vi "GetBandCalculation.vi"(8 "error in (no error)":errorcluster, 11 "Properties In":T2[](array[typedef])) -> (0 "error out":errorcluster, 2 "Calculation":T1, 3 "Properties Out":T2[](array[typedef]))   [LabVIEW 2017, in "AnalysisHelper.lvlib"]
uses:
  <vilib>/addons/InsightCM/Utilities/Analysis/Shared/AnalysisHelper.lvlib
  <vilib>/addons/InsightCM/MessageBus/Base/controls/KeyValuePair.ctl
  <vilib>/addons/InsightCM/Utilities/Analysis/Shared/controls/BandCalculation.ctl
  <vilib>/addons/InsightCM/Utilities/PropertyHelpers/PropertyHelpers.lvlib
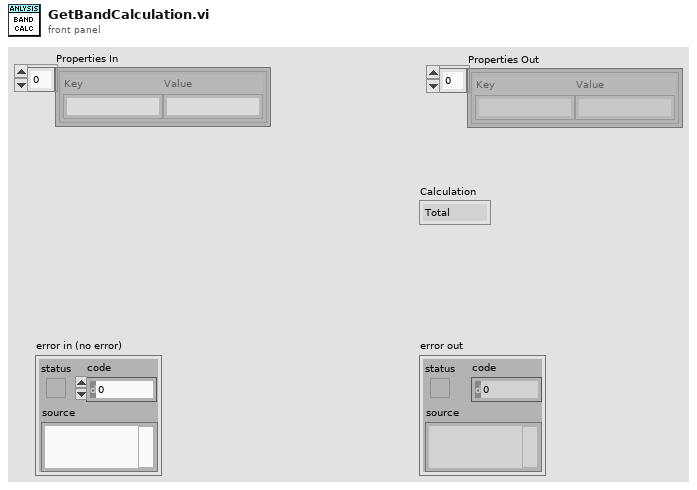
[diagram p1: front panel]
types:
  T1 = typedef "AnalysisHelper.lvlib/BandCalculation.ctl" = enum16{"Total", "Max", "Phase"}
  T2 = typedef "KeyValuePair.ctl" = cluster{"Key":string, "Value":string}
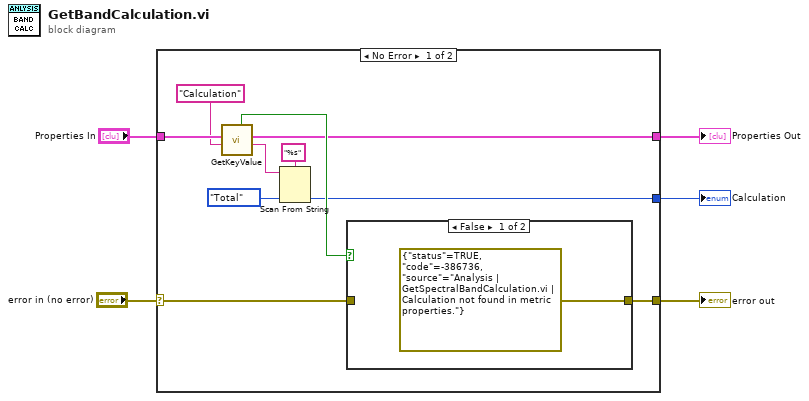
[diagram p0: block diagram]
diagram:
  n1 = case shown="No Error" "error in (no error)" {
    selector: "error in (no error)" -> [w14 w19]
    tunnel: [w8 w18] -> w5
    tunnel: [w11 _] -> w1
    tunnel: "Properties In" -> [w9 w18]
    tunnel: [w15 w19] -> w2
    frame No Error {
      n2 = call <vilib>:"GetKeyValue.vi"("key"="Calculation", "key value pairs"=w9) -> ("value"=w6:string, "key value pairs out"=w8:T2[], "found"=w13:bool)  [unwired: 7 in]
      n3 = Scan From String(format string="%s", input string=w6, default 1=BandCalculation."Total" ("Band Calc")) -> (output 1=w11:T1)  [unwired: 2 in, 3 out]
      n4 = case shown="False" w13 {
        tunnel: [errorcluster {"status"=TRUE, "code"=-386736, "source"="Analysis | GetSpectralBandCalculation.vi | Calculation not found in metric properties."} ("error in") w17] -> w15
        tunnel: w14 -> [_ w17]
        frame False {
        }
        frame True {
        }
      }
    }
    frame Error {
    }
  }
  "Properties Out" <- w5
  "error out" <- w2
  "Calculation" <- w1
